vi "Test Stitch Together Images.vi"() -> ()   [LabVIEW 2011]
uses:
  Type Definitions/Physical Image.ctl
  Vec3d Class/Vec3d Class.lvclass
  <vilib>/vision/Image Controls.llb/IMAQ Image.ctl
  Gantry Class/Gantry Class.lvclass
panel:
  out "Composite Center":cluster{"X":dbl, "Y":dbl, "Z":dbl}
  out "Composite FOV":cluster{"x(mm)":dbl, "y(mm)":dbl}
  in  "Stop":bool
  in  "Grab Image":bool
  out "Preview":T1(plugin-control)
  out "Composite Image":T1(plugin-control)
  in  "Config Folder":path=path "C:/Users/Husker/Desktop/gantry/Config"
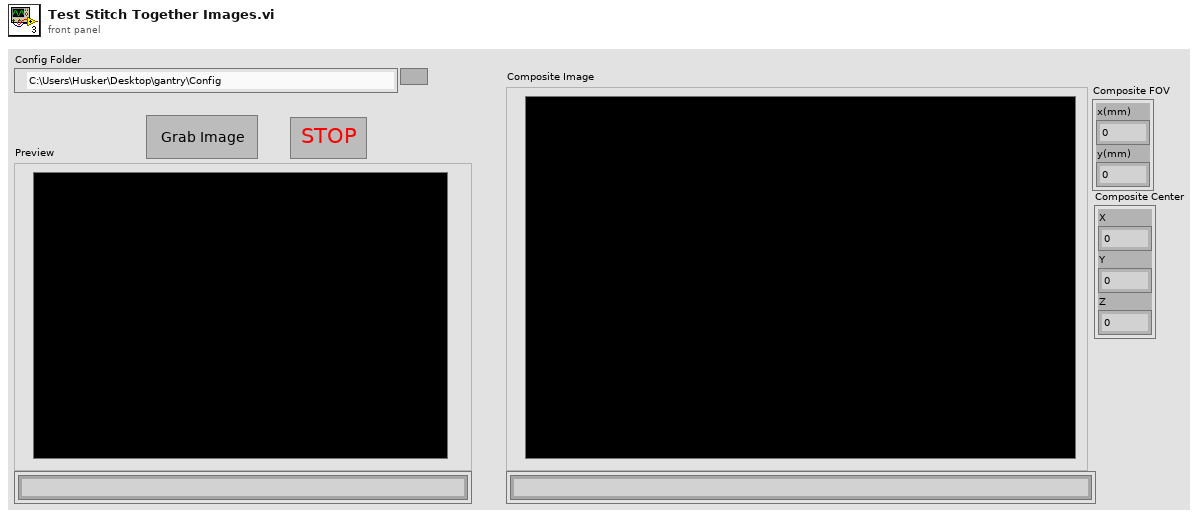
[diagram p1: front panel]
types:
  T1 = typedef "IMAQ Image.ctl" = refnum<image>
  T2 = typedef "Physical Image.ctl" = cluster{"Image Position":refnum<class "Vec3d Class.lvclass">, "Image Reference":T1, "Field of View":cluster{"x(mm)":dbl, "y(mm)":dbl}}
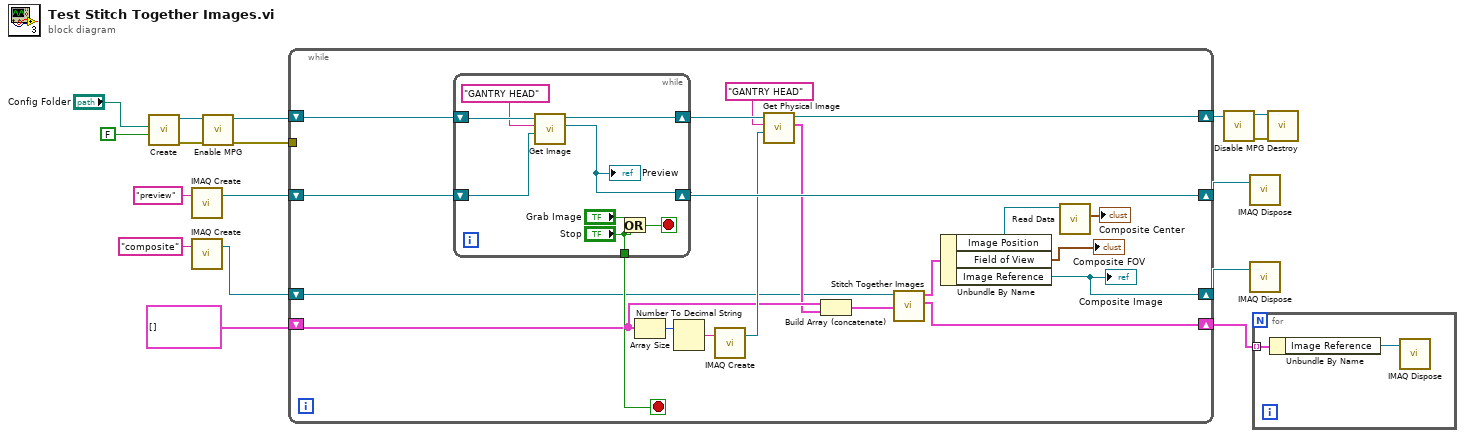
[diagram p0: block diagram]
diagram:
  n1 = call "Create.vi"("HOME?"=FALSE, "Config Folder"="Config Folder") -> ("error out"=w14:errorcluster, "Gantry out"=w15:refnum<class "Gantry Class.lvclass">)  [unwired: 8 in]
  n2 = call "IMAQ Create"("Image Name"="preview") -> ("New Image"=w9:T1)  [unwired: 4 in, 1 out]
  n3 = call "IMAQ Create"("Image Name"="composite") -> ("New Image"=w4:T1)  [unwired: 4 in, 1 out]
  n4 = call-dynamic "Enable MPG.vi"("error in (no error)"=w14, "Gantry Class in"=w15) -> ("error out"=w12:errorcluster, "Gantry Class out"=w13:refnum<class "Gantry Class.lvclass">)  [unwired: 8 in]
  n5 = while {
    tunnel: w12 -> [_]
    shift-right: [w35] -> w2
    shift-left: w9 -> [w36]
    shift-right: [w28] -> w7
    shift-left: w13 -> [w37]
    shift-right: [w21] -> w1
    shift-left: w4 -> [w24]
    shift-right: [w23] -> w3
    shift-left: T2[] [] -> [w27]
    stop <- w34 stop-if-true
    n6 = while {
      shift-right: [w42] -> w35
      shift-left: w36 -> [w43]
      shift-right: [w41] -> w33
      shift-left: w37 -> [w45]
      tunnel: ["Stop"] -> w34
      stop <- w39 stop-if-true
      n7 = call-dynamic "Get Image.vi"("Image In"=w43, "Camera Name"="GANTRY HEAD", "Gantry in"=w45) -> ("Image Out"=w42:T1, "Gantry out"=w41:refnum<class "Gantry Class.lvclass">)  [unwired: 5 in, 2 out]
      "Preview" <- w42
      n8 = Or(x="Grab Image", y="Stop") -> (x .or. y?=w39:bool)
    }
    n9 = Array Size(array=w27) -> (size(s)=w31:i32)
    n10 = Number To Decimal String(number=w31) -> (decimal integer string=w30:string)  [unwired: 1 in]
    n11 = call "IMAQ Create"("Image Name"=w30) -> ("New Image"=w29:T1)  [unwired: 4 in, 1 out]
    n12 = call-dynamic "Get Physical Image.vi"("Image In"=w29, "Camera Name"="GANTRY HEAD", "Gantry in"=w33) -> ("Physical Image"=w26:T2, "Gantry out"=w28:refnum<class "Gantry Class.lvclass">)  [unwired: 6 in, 1 out]
    n13 = Build Array (concatenate)(w27, w26) -> (w25:T2[])
    n14 = call "Stitch Together Images.vi"("Physical Images in"=w25, "Composite Image in"=w24) -> ("Physical Images out"=w23:T2[], "Composite Physical Image"=w22:T2)  [unwired: 7 in, 1 out]
    n15 = Unbundle By Name(w22) -> ("Image Position"=w19:refnum<class "Vec3d Class.lvclass">, "Field of View"=→"Composite FOV":cluster{"x(mm)":dbl, "y(mm)":dbl}, "Image Reference"=w21:T1)
    "Composite Image" <- w21
    n16 = call-dynamic "Read Data.vi"("Vec3d Class in"=w19) -> ("Data"=→"Composite Center":cluster{"X":dbl, "Y":dbl, "Z":dbl})  [unwired: 8 in, 2 out]
  }
  n17 = call-dynamic "Disable MPG.vi"("Gantry Class in"=w7) -> ("error out"=w6:errorcluster, "Gantry Class out"=w5:refnum<class "Gantry Class.lvclass">)  [unwired: 9 in]
  n18 = call "IMAQ Dispose"("Image"=w2) -> ()  [unwired: 5 in, 1 out]
  n19 = call "IMAQ Dispose"("Image"=w1) -> ()  [unwired: 5 in, 1 out]
  n20 = for {
    tunnel: w3 -> [w47] mode=indexing
    n21 = Unbundle By Name(w47) -> ("Image Reference"=w46:T1)
    n22 = call "IMAQ Dispose"("Image"=w46) -> ()  [unwired: 5 in, 1 out]
  }
  n23 = call "Destroy.vi"("error in"=w6, "Gantry Class in"=w5) -> ()  [unwired: 9 in, 1 out]
